vi "APC_9049_CombCluster2Array.vi"(0 "SystemPressure":dbl format="%0.2f", 1 "CombustionAnalysisCluster":T2={"IMEPn [bar]"=[nan, nan, nan, nan, nan, nan], "IMEPg [bar]"=[nan, nan, nan, nan, nan, nan], "MAPO [bar/CAD]"=[nan, nan, nan, nan, nan, nan], "maxQ [J]"=[nan, nan, nan, nan, nan, nan], "CA10  [CADATDC]"=[nan, nan, nan, nan, nan, nan], "CA50 [CADATDC]"=[nan, nan, nan, nan, nan, nan], "CA90 [CADATDC]"=[nan, nan, nan, nan, nan, nan], "Pmax [bar]"=[nan, nan, nan, nan, nan, nan], "IMEPstd [bar]"=[nan, nan, nan, nan, nan, nan], "CA03  [CADATDC]"=[nan, nan, nan, nan, nan, nan], "CA97  [CADATDC]"=[nan, nan, nan, nan, nan, nan], "CA10CA90 [CADATDC]"=[nan, nan, nan, nan, nan, nan], "maxdpdCAD [bar/CAD]"=[nan, nan, nan, nan, nan, nan], "kappa_comp [-]"=[nan, nan, nan, nan, nan, nan], "kappa_exp [-]"=[nan, nan, nan, nan, nan, nan], "PMEP [bar]"=[nan, nan, nan, nan, nan, nan], "RI [-]"=[nan, nan, nan, nan, nan, nan]}, 2 "ExhPressure":dbl format="%0.2f", 3 "PcylDiag":T1[](array[typedef]), 4 "PrechamberPeakPdiff":dbl format="%0.2f") -> (5 "9049_CalculatedVariablesRaster":dbl[](array[numeric]))   [LabVIEW 2020]
uses:
  controls/APC_CombustionMetrics.ctl
  controls/APC_PcylDiag.ctl
panel:
  out "double precision float":dbl[](array[numeric])
  out "WarningsAndErrors":u64[](array[numeric])
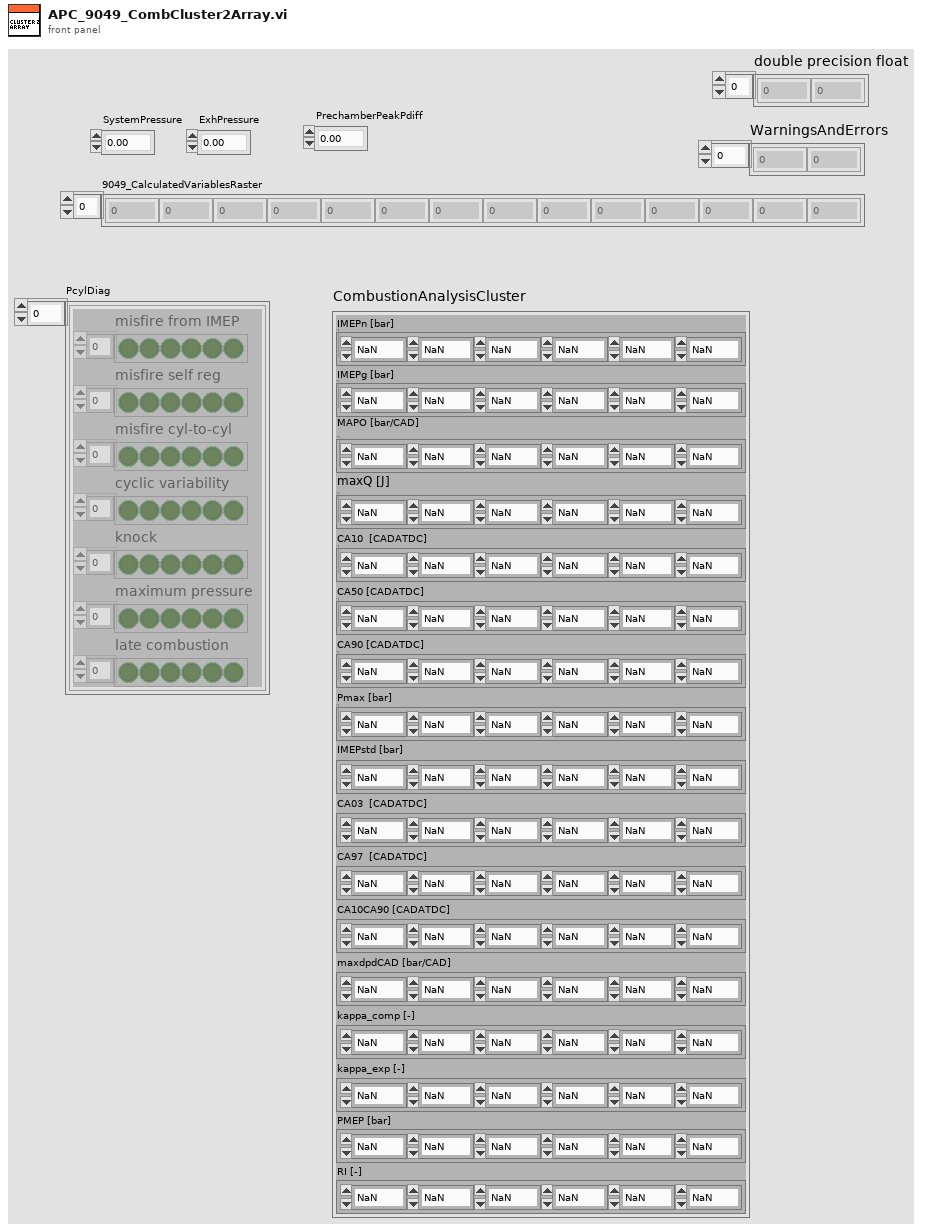
[diagram p1: front panel]
types:
  T1 = typedef "APC_PcylDiag.ctl" = cluster{"misfire from IMEP":bool[], "misfire self reg":bool[], "misfire cyl-to-cyl":bool[], "cyclic variability":bool[], "knock":bool[], "maximum pressure":bool[], "late combustion":bool[]}
  T2 = typedef "APC_CombustionMetrics.ctl" = cluster{"IMEPn [bar]":dbl[], "IMEPg [bar]":dbl[], "MAPO [bar/CAD]":dbl[], "maxQ [J]":dbl[], "CA10  [CADATDC]":dbl[], "CA50 [CADATDC]":dbl[], "CA90 [CADATDC]":dbl[], "Pmax [bar]":dbl[], "IMEPstd [bar]":dbl[], "CA03  [CADATDC]":dbl[], "CA97  [CADATDC]":dbl[], "CA10CA90 [CADATDC]":dbl[], "maxdpdCAD [bar/CAD]":dbl[], "kappa_comp [-]":dbl[], "kappa_exp [-]":dbl[], "PMEP [bar]":dbl[], "RI [-]":dbl[]}
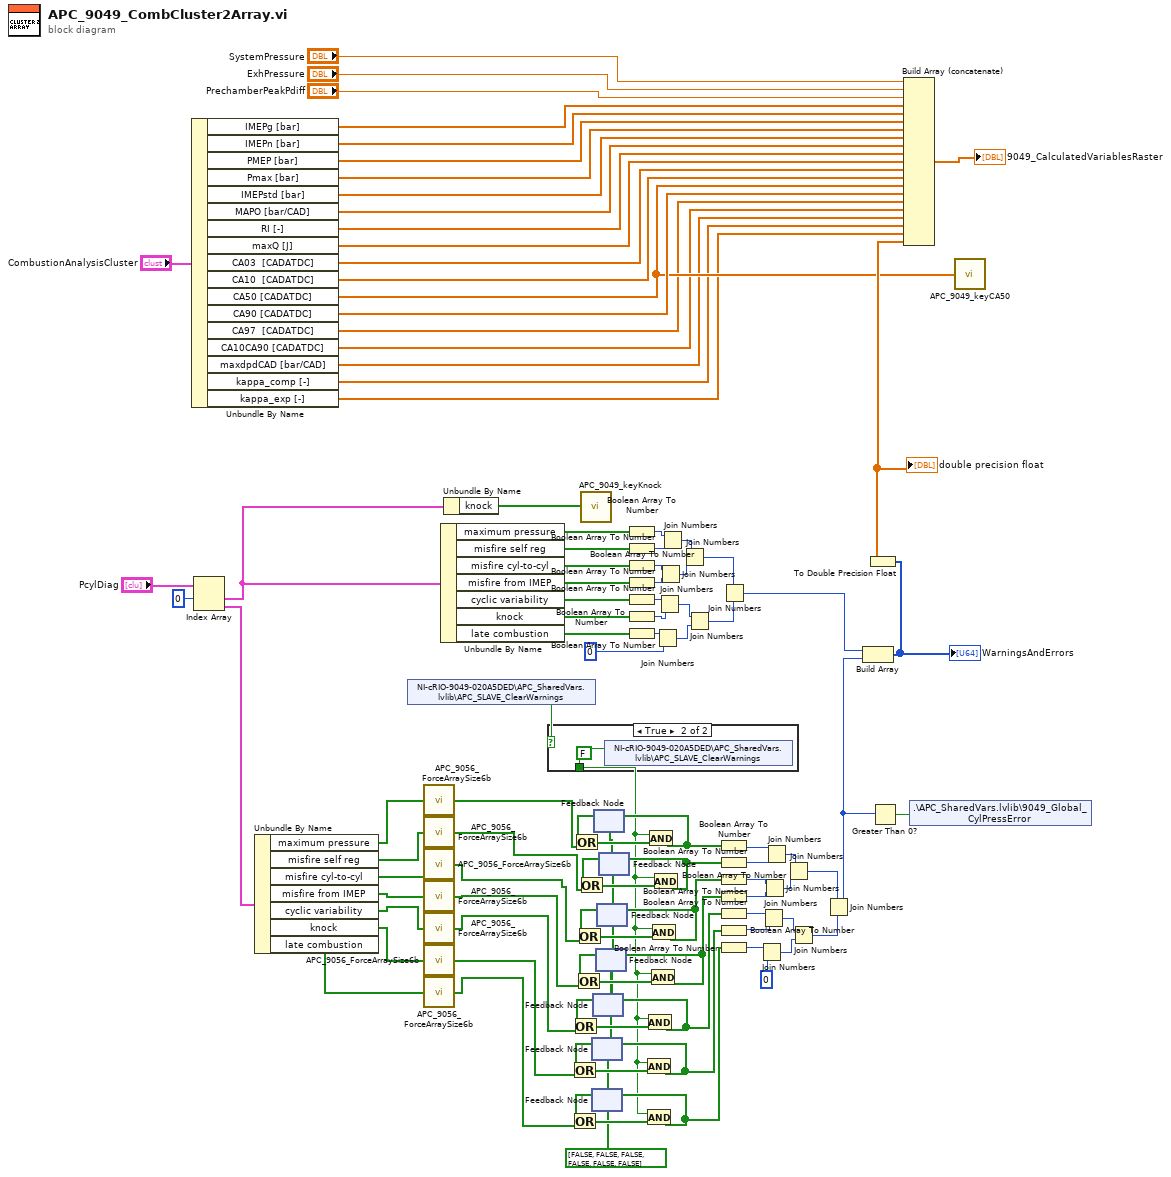
[diagram p0: block diagram]
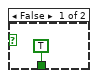
[diagram p2: hidden frame]
diagram:
  w26 = bool[] [FALSE, FALSE, FALSE, FALSE, FALSE, FALSE]
  n1 = Unbundle By Name("CombustionAnalysisCluster") -> ("IMEPg [bar]"=w98:dbl[], "IMEPn [bar]"=w103:dbl[], "PMEP [bar]"=w25:dbl[], "Pmax [bar]"=w99:dbl[], "IMEPstd [bar]"=w100:dbl[], "MAPO [bar/CAD]"=w97:dbl[], "RI [-]"=w24:dbl[], "maxQ [J]"=w96:dbl[], "CA03  [CADATDC]"=w23:dbl[], "CA10  [CADATDC]"=w95:dbl[], "CA50 [CADATDC]"=w92:dbl[], "CA90 [CADATDC]"=w94:dbl[], "CA97  [CADATDC]"=w22:dbl[], "CA10CA90 [CADATDC]"=w21:dbl[], "maxdpdCAD [bar/CAD]"=w20:dbl[], "kappa_comp [-]"=w19:dbl[], "kappa_exp [-]"=w18:dbl[])
  n2 = Index Array(array="PcylDiag", index #1=0 ("index")) -> (element #1=w48:T1, element #2=w68:T1)  [unwired: 1 in]
  n3 = Unbundle By Name(w68) -> ("maximum pressure"=w15:bool[], "misfire self reg"=w14:bool[], "misfire cyl-to-cyl"=w13:bool[], "misfire from IMEP"=w12:bool[], "cyclic variability"=w11:bool[], "knock"=w10:bool[], "late combustion"=w9:bool[])
  n4 = shared-variable "NI-cRIO-9049-020A5DED\\APC_SharedVars.lvlib\\APC_SLAVE_ClearWarnings"() -> (w46:bool)  [unwired: 1 in, 1 out]
  n5 = call "APC_9056_ForceArraySize6b.vi"("ArrayIn"=w15) -> ("ArrayOut"=w8:bool[])
  n6 = call "APC_9056_ForceArraySize6b.vi"("ArrayIn"=w14) -> ("ArrayOut"=w7:bool[])
  n7 = call "APC_9056_ForceArraySize6b.vi"("ArrayIn"=w13) -> ("ArrayOut"=w6:bool[])
  n8 = call "APC_9056_ForceArraySize6b.vi"("ArrayIn"=w12) -> ("ArrayOut"=w5:bool[])
  n9 = call "APC_9056_ForceArraySize6b.vi"("ArrayIn"=w11) -> ("ArrayOut"=w4:bool[])
  n10 = call "APC_9056_ForceArraySize6b.vi"("ArrayIn"=w10) -> ("ArrayOut"=w3:bool[])
  n11 = call "APC_9056_ForceArraySize6b.vi"("ArrayIn"=w9) -> ("ArrayOut"=w2:bool[])
  n12 = Unbundle By Name(w48) -> ("maximum pressure"=w90:bool[], "misfire self reg"=w89:bool[], "misfire cyl-to-cyl"=w88:bool[], "misfire from IMEP"=w87:bool[], "cyclic variability"=w86:bool[], "knock"=w85:bool[], "late combustion"=w84:bool[])
  n13 = Unbundle By Name(w48) -> ("knock"=w47:bool[])
  n14 = case shown="True" w46 {
    tunnel: [TRUE w107] -> w27
    frame False {
    }
    frame True {
      w107 = FALSE
      n15 = shared-variable "NI-cRIO-9049-020A5DED\\APC_SharedVars.lvlib\\APC_SLAVE_ClearWarnings"(w107) -> ()  [unwired: 1 in, 1 out]
    }
  }
  n16 = call "APC_9049_keyKnock.vi"("Knock"=w47) -> ()
  n17 = feedback #1(w26) -> (w37:bool[])
  n18 = Or(x=w37, y=w3) -> (x .or. y?=w36:bool[])
  n19 = feedback #2(w26) -> (w35:bool[])
  n20 = Or(x=w35, y=w2) -> (x .or. y?=w34:bool[])
  n21 = feedback #3(w26) -> (w39:bool[])
  n22 = Or(x=w39, y=w4) -> (x .or. y?=w38:bool[])
  n23 = feedback #4(w26) -> (w51:bool[])
  n24 = Or(x=w51, y=w8) -> (x .or. y?=w50:bool[])
  n25 = feedback #5(w26) -> (w41:bool[])
  n26 = Or(x=w41, y=w5) -> (x .or. y?=w40:bool[])
  n27 = feedback #6(w26) -> (w43:bool[])
  n28 = Or(x=w43, y=w6) -> (x .or. y?=w42:bool[])
  n29 = feedback #7(w26) -> (w45:bool[])
  n30 = Or(x=w45, y=w7) -> (x .or. y?=w44:bool[])
  n31 = Boolean Array To Number(Boolean array=w90) -> (number=w82:u8)
  n32 = Boolean Array To Number(Boolean array=w89) -> (number=w83:u8)
  n33 = Boolean Array To Number(Boolean array=w88) -> (number=w81:u8)
  n34 = Boolean Array To Number(Boolean array=w87) -> (number=w80:u8)
  n35 = Boolean Array To Number(Boolean array=w86) -> (number=w79:u8)
  n36 = Boolean Array To Number(Boolean array=w85) -> (number=w78:u8)
  n37 = Boolean Array To Number(Boolean array=w84) -> (number=w77:u8)
  n38 = And(x=w27, y=w36) -> (x .and. y?=w32:bool[])
  n39 = feedback-in #1(w32) -> ()
  n40 = And(x=w27, y=w34) -> (x .and. y?=w33:bool[])
  n41 = feedback-in #2(w33) -> ()
  n42 = And(x=w27, y=w38) -> (x .and. y?=w31:bool[])
  n43 = feedback-in #3(w31) -> ()
  n44 = And(x=w27, y=w50) -> (x .and. y?=w49:bool[])
  n45 = feedback-in #4(w49) -> ()
  n46 = And(x=w27, y=w40) -> (x .and. y?=w30:bool[])
  n47 = feedback-in #5(w30) -> ()
  n48 = And(x=w27, y=w42) -> (x .and. y?=w28:bool[])
  n49 = feedback-in #6(w28) -> ()
  n50 = And(x=w27, y=w44) -> (x .and. y?=w29:bool[])
  n51 = feedback-in #7(w29) -> ()
  n52 = Join Numbers(hi=w77, lo=u8 0) -> ((hi.lo)=w72:u16)
  n53 = Join Numbers(hi=w79, lo=w78) -> ((hi.lo)=w73:u16)
  n54 = Join Numbers(hi=w81, lo=w80) -> ((hi.lo)=w74:u16)
  n55 = Join Numbers(hi=w82, lo=w83) -> ((hi.lo)=w75:u16)
  n56 = Join Numbers(hi=w75, lo=w74) -> ((hi.lo)=w71:u32)
  n57 = Join Numbers(hi=w73, lo=w72) -> ((hi.lo)=w70:u32)
  n58 = Boolean Array To Number(Boolean array=w49) -> (number=w66:u8)
  n59 = Boolean Array To Number(Boolean array=w29) -> (number=w67:u8)
  n60 = Boolean Array To Number(Boolean array=w28) -> (number=w65:u8)
  n61 = Boolean Array To Number(Boolean array=w30) -> (number=w64:u8)
  n62 = Boolean Array To Number(Boolean array=w31) -> (number=w63:u8)
  n63 = Boolean Array To Number(Boolean array=w32) -> (number=w62:u8)
  n64 = Boolean Array To Number(Boolean array=w33) -> (number=w61:u8)
  n65 = Join Numbers(hi=w71, lo=w70) -> ((hi.lo)=w53:u64)
  n66 = Join Numbers(hi=w61, lo=u8 0) -> ((hi.lo)=w56:u16)
  n67 = Join Numbers(hi=w63, lo=w62) -> ((hi.lo)=w57:u16)
  n68 = Join Numbers(hi=w65, lo=w64) -> ((hi.lo)=w58:u16)
  n69 = Join Numbers(hi=w66, lo=w67) -> ((hi.lo)=w59:u16)
  n70 = Join Numbers(hi=w59, lo=w58) -> ((hi.lo)=w55:u32)
  n71 = Join Numbers(hi=w57, lo=w56) -> ((hi.lo)=w54:u32)
  n72 = Join Numbers(hi=w55, lo=w54) -> ((hi.lo)=w17:u64)
  n73 = Build Array(w53, w17) -> (w52:u64[])
  "WarningsAndErrors" <- w52
  n74 = To Double Precision Float(number=w52) -> (double precision float=w93:dbl[])
  "double precision float" <- w93
  n75 = Greater Than 0?(x=w17) -> (x > 0?=w16:bool)
  n76 = Build Array (concatenate)("SystemPressure", "ExhPressure", "PrechamberPeakPdiff", w98, w103, w25, w99, w100, w97, w24, w96, w23, w95, w92, w94, w22, w21, w20, w19, w18, w93) -> (→"9049_CalculatedVariablesRaster":dbl[])
  n77 = shared-variable ".\\APC_SharedVars.lvlib\\9049_Global_CylPressError"(w16) -> ()  [unwired: 1 in, 1 out]
  n78 = call "APC_9049_keyCA50.vi"("CA50"=w92) -> ()
